vi "Send Voltage.vi"(8 "error in":errorcluster, 11 "69X_79X in":refnum<class "69X_79X.lvclass">) -> (0 "error out":errorcluster, 3 "69X_79X out":refnum<class "69X_79X.lvclass">)   [LabVIEW 2019, in "69X_79X.lvlib" / "69X_79X.lvclass"]
uses:
  Library/69X_79X.lvclass
  C:/Users/Public/Documents/Development/builds/Instruments/PowerSupply.lvlibp/Library/PowerSupply.lvclass
  Accessors/Read Local Resource.vi
  Accessors/Write Local Resource.vi
  <instrlib>/Agilent N6900 N7900 Series/Agilent N6900 N7900 Series.lvlib
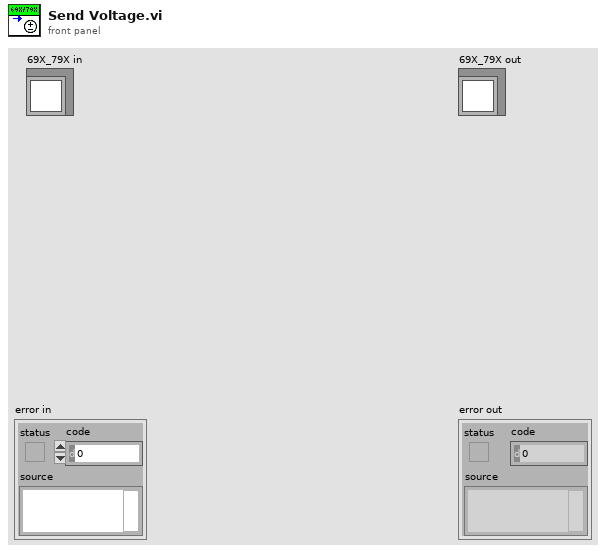
[diagram p1: front panel]
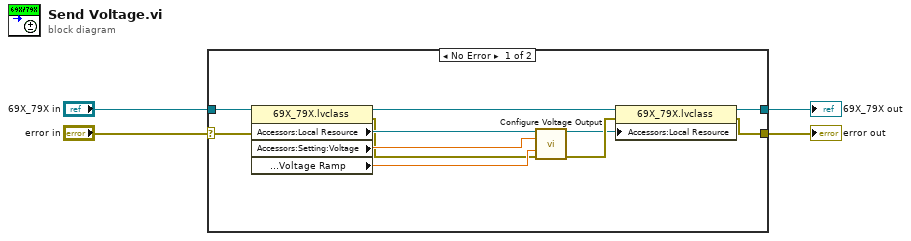
[diagram p0: block diagram]
diagram:
  n1 = case shown="No Error" "error in" {
    selector: "error in" -> [w14 w17]
    tunnel: "69X_79X in" -> [w15 w16]
    tunnel: [w9 w17] -> w3
    tunnel: [w10 w16] -> w4
    frame No Error {
      n2 = property class="69X_79X.lvclass"(reference=w15, error in=w14) -> (reference out=w13:refnum<class "69X_79X.lvclass">, error out=w5:errorcluster, "Accessors:Local Resource"=w6:refnum<visa-resource-name>, "Accessors:Setting:Voltage"=w8:dbl, "Accessors:Setting:Ramp:Voltage Ramp"=w7:dbl)
      n3 = call <instrlib>:"Configure Voltage Output.vi"("VISA resource name"=w6, "Voltage Immediate Amplitude (0 V)"=w8, "Voltage Slew (Inf)"=w7, "error in (no error)"=w5) -> ("VISA resource name out"=w11:refnum<visa-resource-name>, "error out"=w12:errorcluster)  [unwired: 10 in]
      n4 = property class="69X_79X.lvclass"(reference=w13, error in=w12, "Accessors:Local Resource"=w11) -> (reference out=w10:refnum<class "69X_79X.lvclass">, error out=w9:errorcluster)
    }
    frame Error {
    }
  }
  "error out" <- w3
  "69X_79X out" <- w4
